vi "P4CMD Run Command Line.vi"(5 "expected output size":u32=4096, 6 "optional operation parameters":string, 7 "p4 operation":T1, 8 "error in (no error)":errorcluster, 9 "working dir":path, 10 "standard input":string, 11 "p4 global":string) -> (0 "error out":errorcluster, 1 "command error output":string, 2 "command output":string, 4 "return code":i32)   [LabVIEW 2017, in "NI_SCC_P4CMD.lvlib"]
uses:
  <vilib>/SourceControl/Providers/P4CMD/NI_SCC_P4CMD.lvlib
  <vilib>/SourceControl/Providers/P4CMD/P4CMD Operations.ctl
panel:
  out "p4 command":string
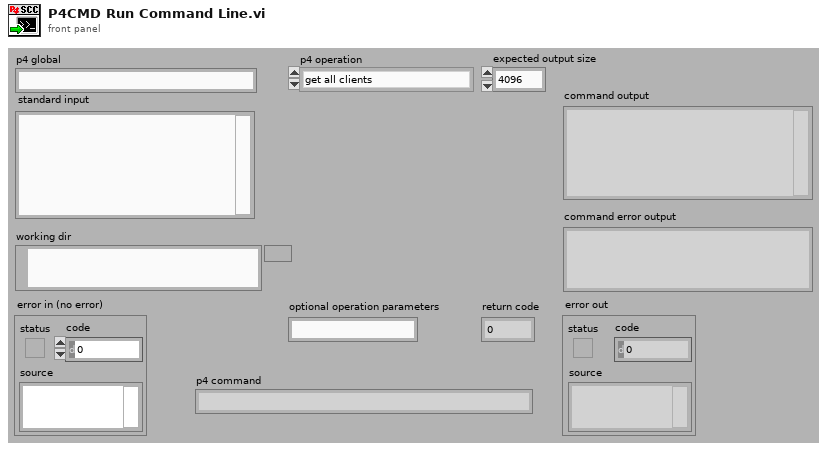
[diagram p1: front panel]
types:
  T1 = typedef "NI_SCC_P4CMD.lvlib/P4CMD Operations.ctl" = enum16{"get all clients", "get all users", "describe changelist", "sync from depot", "open for edit", "submit to depot", "revert", "add to depot", "remove from depot", "print files revisions", "compare client file", "print depot file contents", "list opened files", "get file info", "lock files", "edit changelist spec", "info", "set variables"}
  T2 = enum32{"invalid OS target", "Mac OS", "Windows 3.1", "Windows 95/NT", "Solaris 1", "Solaris 2", "HP-UX", "PowerMAX", "Linux", "Irix", "Rhapsody", "BeOS", "AIX", "OSF1", "VxWorks", "PharLap", "Carbon", "RTX", "Windows x64", "Linux x64", "Mac OS X x64"}
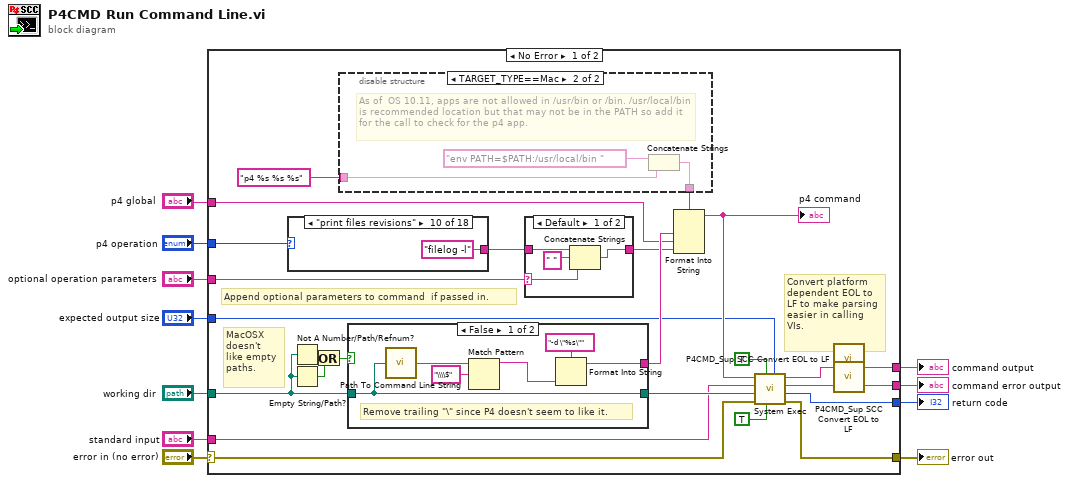
[diagram p0: block diagram]
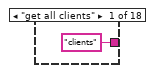
[diagram p4: hidden frame]
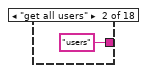
[diagram p5: hidden frame]
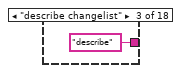
[diagram p6: hidden frame]
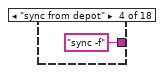
[diagram p7: hidden frame]
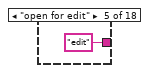
[diagram p8: hidden frame]
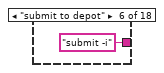
[diagram p9: hidden frame]
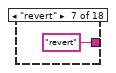
[diagram p10: hidden frame]
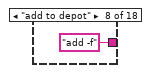
[diagram p11: hidden frame]
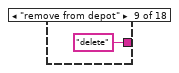
[diagram p12: hidden frame]
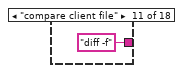
[diagram p13: hidden frame]
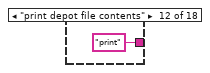
[diagram p14: hidden frame]
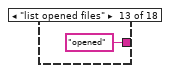
[diagram p15: hidden frame]
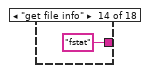
[diagram p16: hidden frame]
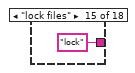
[diagram p17: hidden frame]
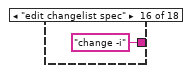
[diagram p18: hidden frame]
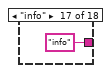
[diagram p19: hidden frame]
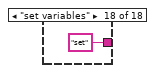
[diagram p20: hidden frame]
diagram:
  n1 = case shown="No Error" "error in (no error)" {
    selector: "error in (no error)" -> [w25 w76]
    tunnel: [w26 w76] -> w10
    tunnel: "p4 global" -> [w24 _]
    tunnel: "working dir" -> [w23 _]
    tunnel: "standard input" -> [w22 _]
    tunnel: [w21 _] -> w6
    tunnel: [w20 _] -> w5
    tunnel: [w17 _] -> w4
    tunnel: "p4 operation" -> [w19 _]
    tunnel: "optional operation parameters" -> [w16 _]
    tunnel: "expected output size" -> [w13 _]
    frame No Error {
      # "Append optional parameters to command  if passed in."
      # "Convert platform dependent EOL to LF to make parsing easier in calling VIs."
      # "MacOSX doesn't\nlike empty paths."
      n2 = case shown="\"print files revisions\"" w19 {
        tunnel: ["clients" ("Format String") "users" ("Format String") "describe" ("string") "sync -f" ("Format String") "edit" ("Format String") "submit -i" ("Format String") "revert" ("Format String") "add -f" ("Format String") "delete" ("Format String") "filelog -l" ("Format String") "diff -f" ("Format String") "print" ("string") "opened" ("Format String") "fstat" ("Format String") "lock" ("Format String") "change -i" ("Format String") "info" ("Format String") "set" ("Format String")] -> w15
        frame "get all clients" {
        }
        frame "get all users" {
        }
        frame "describe changelist" {
        }
        frame "sync from depot" {
        }
        frame "open for edit" {
        }
        frame "submit to depot" {
        }
        frame "revert" {
        }
        frame "add to depot" {
        }
        frame "remove from depot" {
        }
        frame "print files revisions" {
        }
        frame "compare client file" {
        }
        frame "print depot file contents" {
        }
        frame "list opened files" {
        }
        frame "get file info" {
        }
        frame "lock files" {
        }
        frame "edit changelist spec" {
        }
        frame "info" {
        }
        frame "set variables" {
        }
      }
      n3 = Not A Number/Path/Refnum?(number/path/refnum=w23) -> (NaN/Path/Refnum?=w31:bool)
      n4 = Empty String/Path?(string/path=w23) -> (empty?=w30:bool)
      n5 = Or(x=w31, y=w30) -> (x .or. y?=w29:bool)
      n6 = disable-structure shown="TARGET_TYPE==Mac" {
        disable-tunnel: [w37 w39] -> w33
        disable-tunnel: "p4 %s %s %s" ("Format String") -> [w37 w38]
        frame condition #0 (active) {
        }
        frame condition #1 {
          # "As of  OS 10.11, apps are not allowed in /usr/bin or /bin. /usr/local/bin is recommended location but that may not be in the PATH so add it for the call to check for the p4 app."
          n7 = Concatenate Strings("env PATH=$PATH:/usr/local/bin " ("command line"), w38) -> (w39:string)
        }
      }
      n8 = case shown="False" w29 {
        tunnel: [w68 ""] -> w28
        tunnel: w23 -> [w67 _]
        tunnel: [w67 w72] -> w27
        frame False {
          # "Remove trailing \"\\\" since P4 doesn't seem to like it."
          n9 = call <vilib>:"Path To Command Line String.vi"("path"=w67) -> ("string"=w66:string)
          n10 = Match Pattern(string=w66, regular expression="\\\\$") -> (before substring=w65:string)  [unwired: 4 out]
          n11 = Format Into String(format string="-d \"%s\"" ("Format String"), w65) -> (resulting string=w68:string)  [unwired: 2 in, 1 out]
        }
        frame True {
          n12 = property class="App"() -> ("App.TargetOS"=w70:T2)  [unwired: 2 in, 2 out]
          n13 = case shown="Default" w70 {
            tunnel: ["." ("string") ":" ("string")] -> w71
            frame Default {
            }
            frame "Mac OS" {
            }
          }
          n14 = String To Path(string=w71) -> (path=w72:path)
        }
      }
      n15 = case shown="Default" w16 {
        selector: w16 -> [w41 _]
        tunnel: w15 -> [w42 w45]
        tunnel: [w43 w45] -> w14
        frame Default {
          n16 = Concatenate Strings(w42, " " ("string"), w41) -> (w43:string)
        }
        frame "" {
        }
      }
      n17 = Format Into String(format string=w33, w28, w24, w14) -> (resulting string=w32:string)  [unwired: 2 in, 1 out]
      "p4 command" <- w32
      n18 = call <vilib>:"System Exec.vi"("expected output size  (4096)"=w13, "run minimized? (F)"=TRUE ("Run Minimized?"), "wait until completion? (T)"=TRUE ("Wait until Completion?"), "error in (no error)"=w25, "working directory"=w27, "standard input"=w22, "command line"=w32) -> ("error out"=w26:errorcluster, "return code"=w17:i32, "standard error"=w18:string, "standard output"=w34:string)  [unwired: 1 out]
      n19 = call <vilib>:"P4CMD_Sup SCC Convert EOL to LF.vi"("input string"=w34) -> ("output string"=w21:string)  [unwired: 2 out]
      n20 = call <vilib>:"P4CMD_Sup SCC Convert EOL to LF.vi"("input string"=w18) -> ("output string"=w20:string)  [unwired: 2 out]
    }
    frame Error {
    }
  }
  "error out" <- w10
  "command error output" <- w5
  "command output" <- w6
  "return code" <- w4
